vi "Hitronics Get Pump Current.vi"(5 "error in (no error)":errorcluster) -> (14 "Pump Current":dbl, 17 "Full Scan":string, 18 "Continue Exec?":bool, 19 "error out":errorcluster)   [LabVIEW 2020]
panel:
  in  "STOP":bool
  in  "Raw Scan":string
  # "Please insert the Pump Current (A), then hit the <ENTER> key"
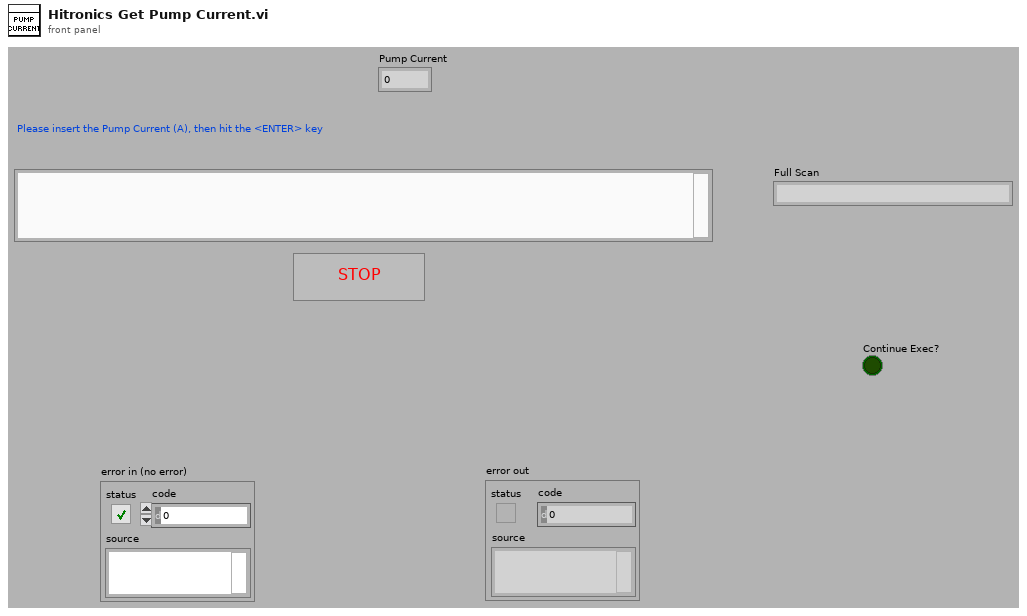
[diagram p1: front panel]
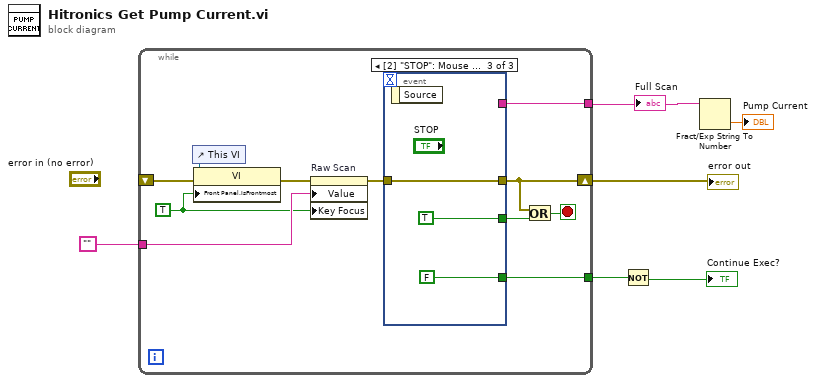
[diagram p0: block diagram]
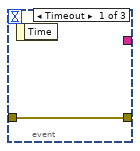
[diagram p2: hidden frame]
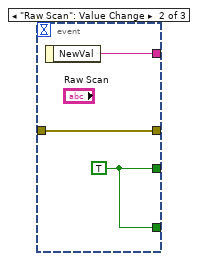
[diagram p3: hidden frame]
diagram:
  n1 = while {
    shift-right: [w17] -> w4
    shift-left: _ -> [w9]
    tunnel: [w14] -> w2
    tunnel: [w13] -> w6
    tunnel: "" -> [w11]
    stop <- w15 stop-if-true
    w7 = TRUE
    n2 = control-ref of="This VI"() -> (w10:refnum<vi>)
    n3 = property class="VI"(reference=w10, error in=w9, "Front Panel.IsFrontmost"=w7) -> (error out=w8:errorcluster)  [unwired: 1 out]
    n4 = property on="Raw Scan" class="Str"(error in=w8, "Value"=w11, "Key Focus"=w7) -> (error out=w12:errorcluster)  [unwired: 1 in, 1 out]
    n5 = event shown="[2] \"STOP\": Mouse Up" {
      selector: _ -> [_ _ _]
      dyn-events: _ -> [_ _ _]
      timeout: _ -> [_ _ _]
      tunnel: w12 -> [w18 w21 w24]
      tunnel: [w18 w21 w24] -> w17
      tunnel: [_ w20 TRUE] -> w16
      tunnel: [_ w20 FALSE] -> w13
      tunnel: [_ w19 _] -> w14
      event Timeout {
        n6 = event-data() -> ()  [unwired: 1 in, 1 out]
      }
      event "Raw Scan": Value Change {
        w20 = TRUE
        n7 = event-data() -> ("NewVal"=w19:string)  [unwired: 1 in]
      }
      event "STOP": Mouse Up {
        n8 = event-data() -> ()  [unwired: 1 in, 1 out]
      }
    }
    n9 = Or(x=w17, y=w16) -> (x .or. y?=w15:bool)
  }
  "error out" <- w4
  "Full Scan" <- w2
  n10 = Not(x=w6) -> (.not. x?=→"Continue Exec?":bool)
  n11 = Fract/Exp String To Number(string=w2) -> (number=→"Pump Current":dbl)  [unwired: 3 in, 1 out]
